vi "Send Response Message.vi"(4 "topic":string, 6 "id":string, 8 "error in":errorcluster, 9 "request error":errorcluster, 10 "result":variant, 11 "Actor Class":T1) -> (0 "error out":errorcluster, 3 "<JSON>Response":string)   [LabVIEW 2019]
uses:
  Actor Private Data.ctl
  <vilib>/LabVIEW Open Source Project/MQTT Client/Client class/Client.lvclass
  Actor Private Events -- cluster.ctl
  Payload -- cluster.ctl
  Response -- cluster.ctl
  3c17847c-a26b-4a8f-b23b-0e08f6d1acdf.vi
  4a429adc-fc73-4a87-8bd2-d85700dce938.vi
  93570760-5aeb-4778-8a40-a1296721cb8c.vi
  <vilib>/JDP Science/JSONtext/Variant to JSON Text.vi
  <vilib>/JDP Science/JSONtext/LVClass Serializer/JSONtext LVClass Serializer.lvclass
  <vilib>/JDP Science/JSONtext/JSONtext.lvlib
  <vilib>/Utility/Data Type/NI_Data Type.lvlib
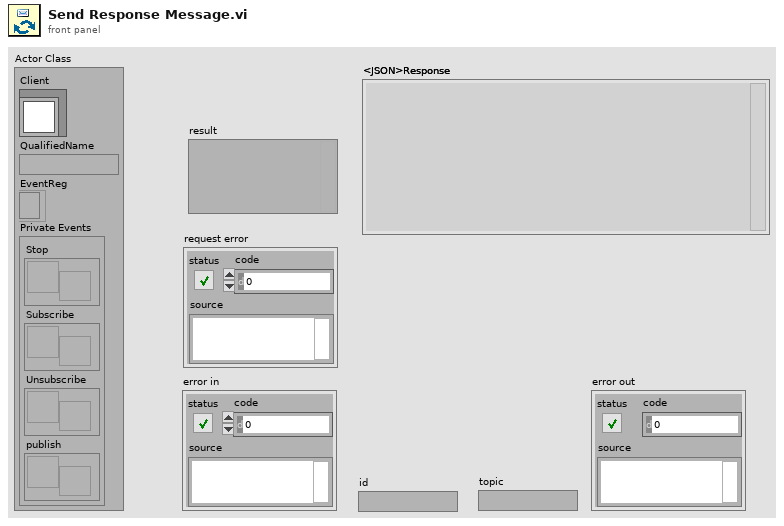
[diagram p1: front panel]
types:
  T1 = typedef "Actor Private Data.ctl" = cluster{"Client":refnum<class "Client.lvclass">, "QualifiedName":string, "EventReg":refnum<event-registration>, "Private Events":T2}
  T2 = typedef "Actor Private Events -- cluster.ctl" = cluster{"Stop":refnum<user-event>, "Subscribe":refnum<user-event>, "Unsubscribe":refnum<user-event>, "publish":refnum<user-event>}
  T3 = typedef "Response -- cluster.ctl" = cluster{"<JSON>result":string, "id":string, "<JSON>error":string}
  T4 = typedef "Payload -- cluster.ctl" = cluster{"topic":string, "Payload":u8[]}
  T5 = typedef "NI_Data Type.lvlib/Data Type.ctl" = enum8{"Invalid Type", "Void", "I8", "I16", "I32", "I64", "U8", "U16", "U32", "U64", "Single Float", "Double Float", "Extended Float", "Single Complex", "Double Complex", "Extended Complex", "Enum U8", "Enum U16", "Enum U32", "Enum U64", "Single Float With Unit", "Double Float With Unit", "Extended Float With Unit", "Single Complex with Unit", "Double Complex with Unit", "Extended Complex with Unit", "Boolean", "String", "Path", "Picture", "Tag", "Array", "Cluster", "Variant", "LV Variant", "Waveform", "Timestamp", "Digital Waveform", "Digital Data", "ExpressData", "Refnum", "External Data", "VI", "Poly VI", "LabVIEW Class Instance", "Fixed Point", "Set Collection", "Map Collection"}
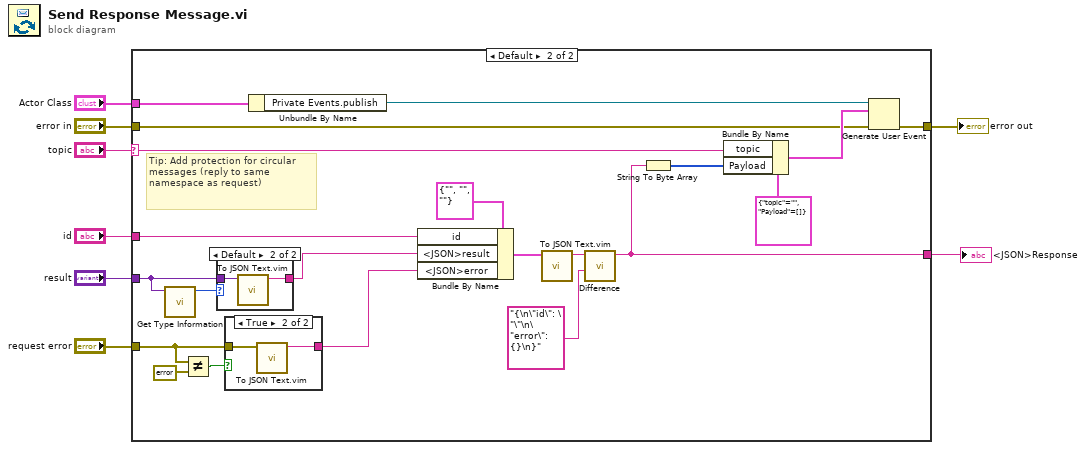
[diagram p0: block diagram]
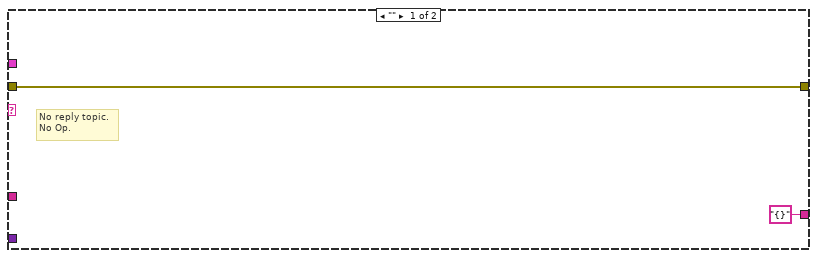
[diagram p2: hidden frame]
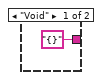
[diagram p3: hidden frame]
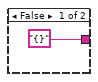
[diagram p4: hidden frame]
diagram:
  n1 = case shown="Default" "topic" {
    selector: "topic" -> [_ w15]
    tunnel: "Actor Class" -> [_ w30]
    tunnel: [w10 w28] -> w7
    tunnel: "error in" -> [w10 w27]
    tunnel: "result" -> [_ w13]
    tunnel: "id" -> [_ w22]
    tunnel: "request error" -> [_ w19]
    tunnel: ["{}" ("<JSON>") w11] -> w1
    frame "" {
      # "No reply topic.\nNo Op."
    }
    frame Default {
      # "Tip: Add protection for circular messages (reply to same namespace as request)"
      n2 = call <vilib>:"Get Type Information.vi"("variant"=w13) -> ("type"=w12:T5)  [unwired: 6 in, 4 out]
      n3 = Not Equal?(x=w19, y=errorcluster {"status"=FALSE, "code"=0, "source"=""} ("request error")) -> (x != y?=w21:bool)
      n4 = case shown="Default" w12 {
        tunnel: ["{}" ("<JSON>") w34] -> w14
        tunnel: w13 -> [_ w33]
        frame "Void" {
        }
        frame Default {
          n5 = call "To JSON Text.vim"("Anything"=w33) -> ("<JSON>"=w34:string)  [unwired: 9 in, 1 out]
        }
      }
      n6 = case shown="True" w21 {
        tunnel: w19 -> [_ w37]
        tunnel: ["{}" ("error") w36] -> w18
        frame False {
        }
        frame True {
          n7 = call "To JSON Text.vim"("Anything"=w37) -> ("<JSON>"=w36:string)  [unwired: 9 in, 1 out]
        }
      }
      n8 = Unbundle By Name(w30) -> ("Private Events.publish"=w26:refnum<user-event>)
      n9 = Bundle By Name(cluster=T3 {"<JSON>result"="", "id"="", "<JSON>error"=""} ("response"), "id"=w22, "<JSON>result"=w14, "<JSON>error"=w18) -> (w24:T3)
      n10 = call "To JSON Text.vim"("Anything"=w24) -> ("<JSON>"=w17:string)  [unwired: 9 in, 1 out]
      n11 = call <vilib>:"Difference.vi"("Compare to this JSON Object"="{\n\"id\": \"\"\n\"error\": {}\n}", "JSON Object"=w17) -> ("<JSON>"=w11:string)  [unwired: 7 in, 1 out]
      n12 = String To Byte Array(string=w11) -> (unsigned byte array=w25:u8[])
      n13 = Bundle By Name(cluster=T4 {"topic"="", "Payload"=[]} ("publish"), "topic"=w15, "Payload"=w25) -> (w29:T4)
      n14 = Generate User Event(user event=w26, event data cluster=w29, error in=w27) -> (error out=w28:errorcluster)  [unwired: 1 in, 1 out]
    }
  }
  "error out" <- w7
  "<JSON>Response" <- w1
